vi "Calculate_DCMotor_Spin.vi"(10 "Wheel Angles":T2={"alpha1"=330.0, "alpha2"=90.0, "alpha3"=210.0}, 11 "Calibrated Oculus Data":T1) -> (1 "M3":dbl, 2 "M2":dbl, 3 "M1":dbl)   [LabVIEW 2017]
uses:
  Calibrated Oculus Data.ctl
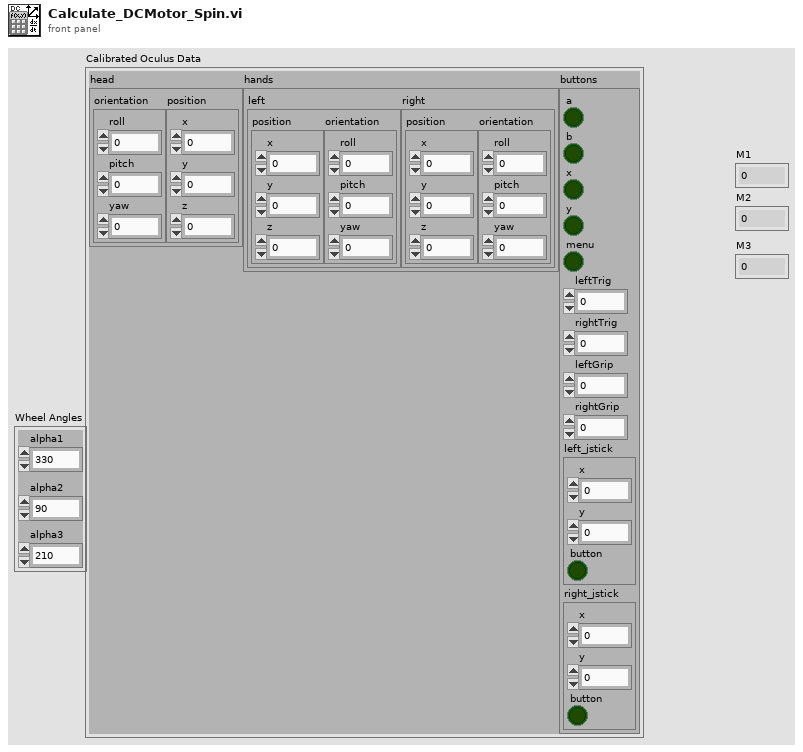
[diagram p1: front panel]
types:
  T1 = typedef "Calibrated Oculus Data.ctl" = cluster{"head":cluster{"orientation":cluster{"roll":dbl, "pitch":dbl, "yaw":dbl}, "position":cluster{"x":dbl, "y":dbl, "z":dbl}}, "hands":cluster{"left":cluster{"position":cluster{"x":dbl, "y":dbl, "z":dbl}, "orientation":cluster{"roll":dbl, "pitch":dbl, "yaw":dbl}}, "right":cluster{"position":cluster{"x":dbl, "y":dbl, "z":dbl}, "orientation":cluster{"roll":dbl, "pitch":dbl, "yaw":dbl}}}, "buttons":cluster{"a":bool, "b":bool, "x":bool, "y":bool, "menu":bool, "leftTrig":dbl, "rightTrig":dbl, "leftGrip":dbl, "rightGrip":dbl, "left_jstick":cluster{"x":dbl, "y":dbl, "button":bool}, "right_jstick":cluster{"x":dbl, "y":dbl, "button":bool}}}
  T2 = cluster{"alpha1":dbl, "alpha2":dbl, "alpha3":dbl}
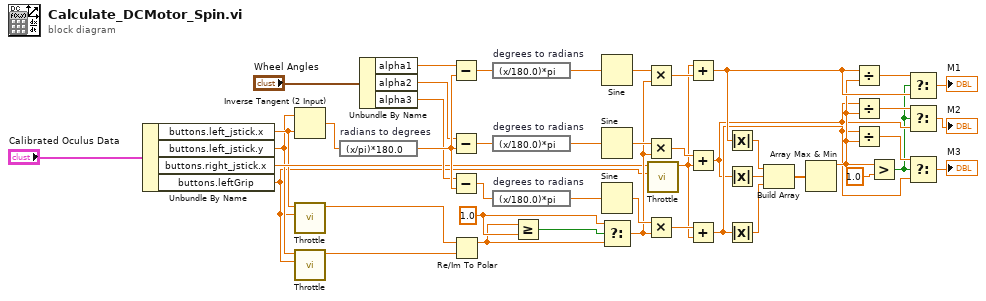
[diagram p0: block diagram]
diagram:
  w33 = 1.0 ("t")
  n1 = Unbundle By Name("Calibrated Oculus Data") -> ("buttons.left_jstick.x"=w6:dbl, "buttons.left_jstick.y"=w4:dbl, "buttons.right_jstick.x"=w7:dbl, "buttons.leftGrip"=w3:dbl)
  n2 = Inverse Tangent (2 Input)(1:w6, 2:w4) -> (0:w46:dbl)
  n3 = call "Throttle.vi"("Throttle"=w3, "Input"=w6) -> ("Output"=w5:dbl)  [unwired: 9 in]
  n4 = call "Throttle.vi"("Throttle"=w3, "Input"=w4) -> ("Output"=w2:dbl)  [unwired: 9 in]
  n5 = expression code="(x/pi)*180.0" "radians to degrees"(w46) -> (w45:dbl)
  n6 = Unbundle By Name("Wheel Angles") -> ("alpha1"=w11:dbl, "alpha2"=w10:dbl, "alpha3"=w9:dbl)
  n7 = Subtract(x=w11, y=w45) -> (x-y=w42:dbl)
  n8 = Subtract(x=w10, y=w45) -> (x-y=w44:dbl)
  n9 = Subtract(x=w9, y=w45) -> (x-y=w43:dbl)
  n10 = Re/Im To Polar(2:w2, 3:w5) -> (1:w13:dbl)  [unwired: 1 out]
  n11 = expression code="(x/180.0)*pi" "degrees to radians"(w42) -> (w40:dbl)
  n12 = expression code="(x/180.0)*pi" "degrees to radians"(w44) -> (w38:dbl)
  n13 = expression code="(x/180.0)*pi" "degrees to radians"(w43) -> (w36:dbl)
  n14 = Greater Or Equal?(x=w13, y=w33) -> (x >= y?=w34:bool)
  n15 = Sine(x=w40) -> (sin(x)=w41:dbl)
  n16 = Sine(x=w38) -> (sin(x)=w39:dbl)
  n17 = Sine(x=w36) -> (sin(x)=w37:dbl)
  n18 = Select(t=w33, s=w34, f=w13) -> (s? t:f=w35:dbl)
  n19 = Multiply(x=w41, y=w35) -> (x*y=w32:dbl)
  n20 = Multiply(x=w39, y=w35) -> (x*y=w31:dbl)
  n21 = Multiply(x=w37, y=w35) -> (x*y=w30:dbl)
  n22 = call "Throttle.vi"("Throttle"=w3, "Input"=w7) -> ("Output"=w8:dbl)  [unwired: 9 in]
  n23 = Add(x=w8, y=w32) -> (x+y=w24:dbl)
  n24 = Add(x=w31, y=w8) -> (x+y=w19:dbl)
  n25 = Add(x=w30, y=w8) -> (x+y=w20:dbl)
  n26 = Absolute Value(x=w24) -> (abs(x)=w28:dbl)
  n27 = Absolute Value(x=w19) -> (abs(x)=w27:dbl)
  n28 = Absolute Value(x=w20) -> (abs(x)=w26:dbl)
  n29 = Build Array(w28, w27, w26) -> (w29:dbl[])
  n30 = Array Max & Min(array=w29) -> (max value=w21:dbl)  [unwired: 3 out]
  n31 = Divide(x=w24, y=w21) -> (x/y=w14:dbl)
  n32 = Divide(x=w19, y=w21) -> (x/y=w22:dbl)
  n33 = Divide(x=w20, y=w21) -> (x/y=w23:dbl)
  n34 = Greater?(x=w21, y=1.0) -> (0:w15:bool)
  n35 = Select(t=w14, s=w15, f=w24) -> (s? t:f=→"M1":dbl)
  n36 = Select(t=w22, s=w15, f=w19) -> (s? t:f=→"M2":dbl)
  n37 = Select(t=w23, s=w15, f=w20) -> (s? t:f=→"M3":dbl)
